vi "GE 5565PIORC.DMA.Endianness.vi"(11 "count (1000)":u32=1000) -> (0 "error out":errorcluster, 3 "pass?":bool)   [LabVIEW 2016]
uses:
  <vilib>/NI/GE Reflective Memory Driver/GE 5565PIORC.lvclass/GE 5565PIORC.ctl
  <vilib>/NI/GE Reflective Memory Driver/Methods/GE 5565PIORC.DMA.Block.Write (DBL).vi
  <vilib>/NI/GE Reflective Memory Driver/Methods/GE 5565PIORC.DMA.Create Transfer (Block).vi
  <vilib>/NI/GE Reflective Memory Driver/Methods/GE 5565PIORC.DMA.Block.Read (DBL).vi
  <vilib>/NI/GE Reflective Memory Driver/Properties/Registers/GE 5565PIORC.Registers.DMACSR0.Channel 0 Enable.Set.vi
  <vilib>/NI/GE Reflective Memory Driver/Properties/GE 5565PIORC.Read VISA MEMACC.vi
  <vilib>/NI/GE Reflective Memory Driver/Methods/GE 5565PIORC.DMA.Create Transfer (Scatter-Gather).vi
  <vilib>/NI/GE Reflective Memory Driver/Methods/GE 5565PIORC.DMA.Configure.vi
  <vilib>/NI/GE Reflective Memory Driver/Methods/GE 5565PIORC.PXI Interrupts.Discard Events.vi
  <vilib>/NI/GE Reflective Memory Driver/Methods/GE 5565PIORC.DMA.Start.vi
  <vilib>/NI/GE Reflective Memory Driver/Methods/GE 5565PIORC.DMA.Interrupt.Wait for Done.vi
  <vilib>/NI/GE Reflective Memory Driver/Properties/Registers/GE 5565PIORC.Registers.Local Configuration.Read.vi
  <vilib>/NI/GE Reflective Memory Driver/Properties/Registers/GE 5565PIORC.Registers.Local Configuration.Read (U8).vi
  <vilib>/NI/GE Reflective Memory Driver/Properties/Registers/GE 5565PIORC.Registers.Local Configuration.Write.vi
  <vilib>/NI/GE Reflective Memory Driver/Properties/Registers/GE 5565PIORC.Registers.Local Configuration.Write (U8).vi
  <vilib>/NI/GE Reflective Memory Driver/Methods/GE 5565PIORC.Bit Manipulation.Set Bit.vi
  <vilib>/NI/GE Reflective Memory Driver/Methods/GE 5565PIORC.Bit Manipulation.Set Bit (U8).vi
  <vilib>/NI/GE Reflective Memory Driver/Methods/GE 5565PIORC.DMA.Size.vi
  <vilib>/NI/GE Reflective Memory Driver/Properties/Registers/GE 5565PIORC.Registers.DMADPR0.Direction of Transfer.Set.vi
  <vilib>/NI/GE Reflective Memory Driver/Properties/Registers/GE 5565PIORC.Registers.DMASIZ0.DMA Transfer Size.Set.vi
  <vilib>/NI/GE Reflective Memory Driver/Properties/Registers/GE 5565PIORC.Registers.DMALADR0.Local Address Register.Set.vi
  <vilib>/NI/GE Reflective Memory Driver/Properties/Registers/GE 5565PIORC.Registers.DMAMODE0.Scatter-Gather Mode.Set.vi
  <vilib>/NI/GE Reflective Memory Driver/Properties/Registers/GE 5565PIORC.Registers.DMAPADR0.PCI Address Register.Set.vi
  <vilib>/NI/GE Reflective Memory Driver/Methods/GE 5565PIORC.DMA.Scatter-Gather.Link Block Descriptors.vi
  <vilib>/NI/GE Reflective Memory Driver/Methods/GE 5565PIORC.DMA.Scatter-Gather.Commit Linked Block Descriptors.vi
  <vilib>/NI/GE Reflective Memory Driver/Properties/Registers/GE 5565PIORC.Registers.DMADPR0.Channel 0 First Descriptor Address.Set.vi
  <vilib>/Utility/error.llb/Clear Errors.vi
  <vilib>/NI/GE Reflective Memory Driver/Properties/Registers/GE 5565PIORC.Registers.DMACSR0.Channel 0 Start.Set.vi
  <vilib>/NI/GE Reflective Memory Driver/Methods/GE 5565PIORC.PXI Interrupts.Wait for Event.vi
  <vilib>/NI/GE Reflective Memory Driver/Properties/Registers/GE 5565PIORC.Registers.DMACSR0.Channel 0 Clear Interrupt.Set.vi
  <vilib>/NI/GE Reflective Memory Driver/Methods/GE 5565PIORC.Registers.Read.vi
  <vilib>/NI/GE Reflective Memory Driver/Methods/GE 5565PIORC.Registers.Read (U8).vi
  <vilib>/NI/GE Reflective Memory Driver/Methods/GE 5565PIORC.Registers.Write.vi
  <vilib>/NI/GE Reflective Memory Driver/Methods/GE 5565PIORC.Registers.Write (U8).vi
  <vilib>/NI/GE Reflective Memory Driver/Properties/Registers/GE 5565PIORC.Registers.Local Configuration.Read (U32).vi
  <vilib>/NI/GE Reflective Memory Driver/Properties/Registers/GE 5565PIORC.Registers.Local Configuration.Write (U32).vi
  <vilib>/NI/GE Reflective Memory Driver/Methods/GE 5565PIORC.Bit Manipulation.Set Bit (U32).vi
  <vilib>/NI/GE Reflective Memory Driver/Methods/GE 5565PIORC.DMA.Scatter-Gather.Set Descriptor Params.vi
  <vilib>/NI/GE Reflective Memory Driver/Methods/GE 5565PIORC.Registers.Read (U32).vi
  <vilib>/NI/GE Reflective Memory Driver/Methods/GE 5565PIORC.Registers.Write (U32).vi
  <vilib>/NI/GE Reflective Memory Driver/Methods/GE 5565PIORC.Round Up to Nearest 8.vi
  <vilib>/NI/GE Reflective Memory Driver/Methods/GE 5565PIORC.Round Up to Nearest 16.vi
  <vilib>/NI/GE Reflective Memory Driver/GE 5565PIORC.lvclass
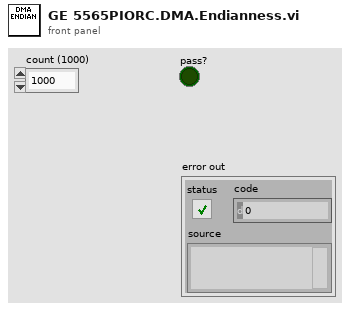
[diagram p1: front panel]
types:
  T1 = enum16{"big-endian, network order", "native, host order", "little-endian"}
  T2 = typedef "GE 5565PIORC.lvclass/GE 5565PIORC.Typedef.DMA Block Descriptor.ctl" = cluster{"descriptor ptr (VISA)":u32, "descriptor ptr (RFM)":u32, "descriptor size":u32, "descriptor params":T3}
  T3 = typedef "GE 5565PIORC.lvclass/GE 5565PIORC.Typedef.DMA Block Descriptor Params.ctl" = cluster{"data ptr (lower)":u32, "data ptr (upper)":u32, "data size":u32, "next descriptor ptr":u32}
  T4 = typedef "GE 5565PIORC.lvclass/GE 5565PIORC.Typedef.DMA Transfer Spec.ctl" = cluster{"RFM offset":u32, "Block Descriptors":T2[]}
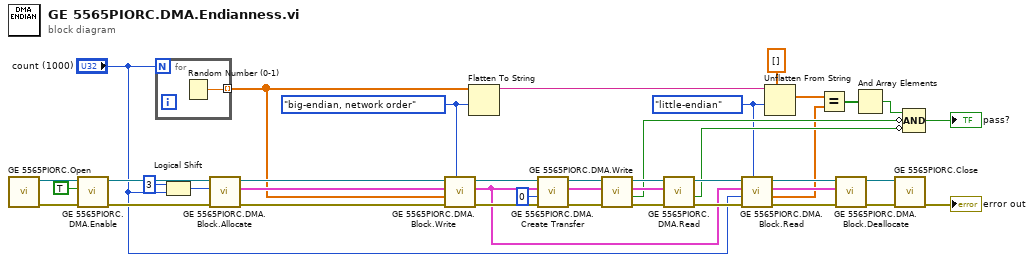
[diagram p0: block diagram]
diagram:
  w2 = T1."big-endian, network order" ("byte order (0:big-endian, network order)")
  w7 = T1."little-endian" ("byte order (0:big-endian, network order)")
  n1 = call "GE 5565PIORC.Open.vi"() -> ("error out"=w9:errorcluster, "GE 5565PIORC"=w10:refnum<class "GE 5565PIORC.lvclass">)  [unwired: 10 in]
  n2 = call <vilib>:"GE 5565PIORC.DMA.Enable.vi"("error in (no error)"=w9, "enable (T)"=TRUE ("Enable DMA"), "GE 5565PIORC in"=w10) -> ("error out"=w38:errorcluster, "GE 5565PIORC out"=w39:refnum<class "GE 5565PIORC.lvclass">)  [unwired: 7 in]
  n3 = for {
    N: "count (1000)" -> [_]
    tunnel: [w42] -> w1 mode=indexing
    n4 = Random Number (0-1)() -> (number: 0 to 1=w42:dbl)
  }
  n5 = Logical Shift(y=i16 3, x="count (1000)") -> (x << y=w33:u32)
  n6 = call <vilib>:"GE 5565PIORC.DMA.Block.Allocate.vi"("error in (no error)"=w38, "size in bytes"=w33, "GE 5565PIORC in"=w39) -> ("error out"=w35:errorcluster, "Block Descriptor"=w34:T2, "GE 5565PIORC out"=w36:refnum<class "GE 5565PIORC.lvclass">)  [unwired: 6 in]
  n7 = call-poly <vilib>:"GE 5565PIORC.DMA.Block.Write.vi"("byte order (big-endian)"=w2, "error in (no error)"=w35, "data"=w1, "Block Descriptor in"=w34, "GE 5565PIORC in"=w36) -> ("error out"=w30:errorcluster, "Block Descriptor out"=w27:T2, "GE 5565PIORC out"=w31:refnum<class "GE 5565PIORC.lvclass">)  [unwired: 3 in, 1 out]
  n8 = Flatten To String(anything=w1, byte order (0:big-endian, network order)=w2) -> (data string=w8:string)  [unwired: 2 in, 2 out]
  n9 = call-poly <vilib>:"GE 5565PIORC.DMA.Create Transfer.vi"("error in (no error)"=w30, "RFM offset"=u32 0, "Block Descriptor"=w27, "GE 5565PIORC in"=w31) -> ("error out"=w16:errorcluster, "DMA Transfer Spec"=w15:T4, "GE 5565PIORC out"=w17:refnum<class "GE 5565PIORC.lvclass">)  [unwired: 4 in, 1 out]
  n10 = call <vilib>:"GE 5565PIORC.DMA.Write.vi"("error in (no error)"=w16, "DMA Transfer Spec"=w15, "GE 5565PIORC in"=w17) -> ("error out"=w12:errorcluster, "timed out?"=w11:bool, "DMA Transfer Spec dup"=w14:T4, "GE 5565PIORC out"=w13:refnum<class "GE 5565PIORC.lvclass">)  [unwired: 5 in]
  n11 = call <vilib>:"GE 5565PIORC.DMA.Read.vi"("error in (no error)"=w12, "DMA Transfer Spec"=w14, "GE 5565PIORC in"=w13) -> ("error out"=w28:errorcluster, "timed out?"=w23:bool, "GE 5565PIORC out"=w29:refnum<class "GE 5565PIORC.lvclass">)  [unwired: 5 in, 1 out]
  n12 = call-poly <vilib>:"GE 5565PIORC.DMA.Block.Read.vi"("byte order (big-endian)"=w7, "error in (no error)"=w28, "count"="count (1000)", "Block Descriptor in"=w27, "GE 5565PIORC in"=w29) -> ("error out"=w24:errorcluster, "data out"=w4:dbl[], "Block Descriptor out"=w25:T2, "GE 5565PIORC out"=w26:refnum<class "GE 5565PIORC.lvclass">)  [unwired: 3 in]
  n13 = Unflatten From String(type=dbl[] [] ("data out"), binary string=w8, byte order (0:big-endian, network order)=w7) -> (value=w5:dbl[])  [unwired: 2 in, 2 out]
  n14 = Equal?(x=w5, y=w4) -> (x = y?=w22:bool[])
  n15 = call <vilib>:"GE 5565PIORC.DMA.Block.Deallocate.vi"("error in (no error)"=w24, "Block Descriptor"=w25, "GE 5565PIORC in"=w26) -> ("error out"=w19:errorcluster, "GE 5565PIORC out"=w20:refnum<class "GE 5565PIORC.lvclass">)  [unwired: 7 in]
  n16 = And Array Elements(Boolean array=w22) -> (logical AND=w21:bool)
  n17 = call "GE 5565PIORC.Close.vi"("error in (no error)"=w19, "GE 5565PIORC"=w20) -> ("error out"=→"error out":errorcluster)  [unwired: 9 in]
  n18 = Compound Arithmetic op=AND(w21, invert w11, invert w23) -> (→"pass?":bool)
